vi "20 Limit 180 Degrees (x64-2018).vi"(1 "Angle In":dynamicdata(waveform)) -> (0 "Angle Out":dynamicdata(waveform))   [LabVIEW 2017]
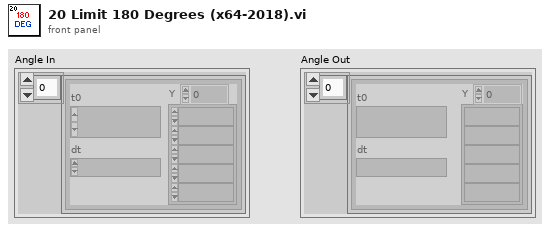
[diagram p1: front panel]
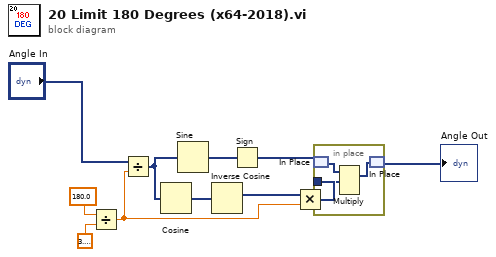
[diagram p0: block diagram]
diagram:
  n1 = Divide(x=180.0, y=3.141592653589793) -> (x/y=w3:dbl)
  n2 = Divide(x="Angle In", y=w3) -> (x/y=w7:dynamicdata)
  n3 = Cosine(x=w7) -> (cos(x)=w6:dynamicdata)
  n4 = Sine(x=w7) -> (sin(x)=w5:dynamicdata)
  n5 = Inverse Cosine(1:w6) -> (0:w4:dynamicdata)
  n6 = Sign(1:w5) -> (0:w2:dynamicdata)
  n7 = Multiply(x=w4, y=w3) -> (x*y=w1:dynamicdata)
  n8 = in-place {
    in-place-border: w1 -> [w12]
    n9 = in-place-match #1(w2) -> (w13:dynamicdata)
    n10 = Multiply(1:w12, 2:w13) -> (0:w14:dynamicdata)  [unwired: 1 in, 1 out]
    n11 = in-place-match #1(w14) -> (→"Angle Out":dynamicdata)
  }
